vi "init_round_buoy.vi"(9 "Mission.lvclass":refnum<class "Mission.lvclass">, 11 "Buoy Round":cluster{"X":dbl, "Y":dbl}) -> (3 "Mission out":refnum<class "Mission.lvclass">)   [LabVIEW 2011, in "Mission.lvclass"]
uses:
  Mission.lvclass
  Mission.lvclass/Mission.ctl
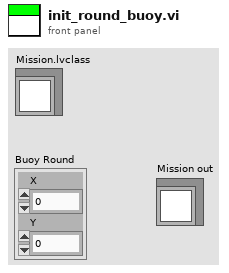
[diagram p1: front panel]
types:
  T1 = enum16{"Round Buoy", "Pass Buoys", "Station Keeping"}
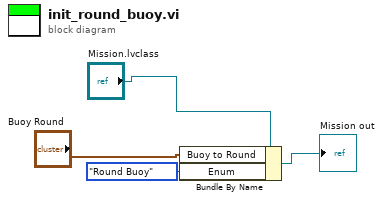
[diagram p0: block diagram]
diagram:
  n1 = Bundle By Name(cluster="Mission.lvclass", "Buoy to Round"="Buoy Round", "Enum"=T1."Round Buoy") -> (→"Mission out":refnum<class "Mission.lvclass">)
